vi "CalculateTotalCharge.vi"(9 "Period (sec)":dbl, 10 "Beam Current (A)":dbl, 11 "Total Charge In (C)":dbl) -> (3 "Total Charge Out (C)":dbl)   [LabVIEW 2012]
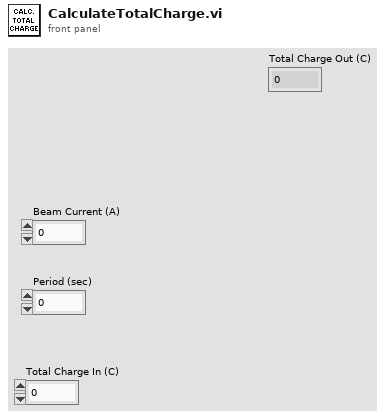
[diagram p1: front panel]
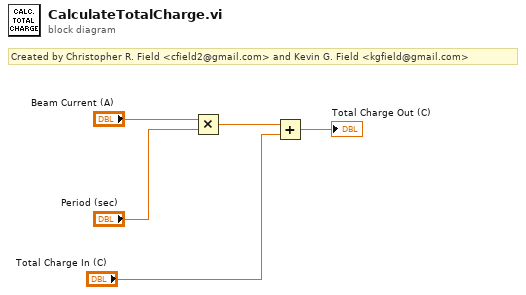
[diagram p0: block diagram]
diagram:
  # "Created by Christopher R. Field <cfield2@gmail.com> and Kevin G. Field <kgfield@gmail.com>"
  n1 = Multiply(x="Beam Current (A)", y="Period (sec)") -> (x*y=w3:dbl)
  n2 = Add(x=w3, y="Total Charge In (C)") -> (x+y=→"Total Charge Out (C)":dbl)
